vi "stop.vi"(8 "error in (no error)":errorcluster, 11 "references":T1) -> (0 "error out":errorcluster)   [LabVIEW 2015, in "lv-recipe-machine.lvlib"]
doc: "stop.vi will stop the asynchronously running main and de-allocate any internal resources."
uses:
  lv-recipe-machine.lvlib
  _controls/references.ctl
  _controls/change.ctl
  _controls/automatic_state.ctl
  _controls/manual_state.ctl
  _controls/mode.ctl
  _controls/status.ctl
  _controls/configuration.ctl
  _controls/recipe_step.ctl
  _controls/recipe_data.ctl
  _controls/data.ctl
  _controls/output.ctl
  _controls/input_command.ctl
  _controls/input.ctl
  _controls/transition.ctl
  _controls/timer.ctl
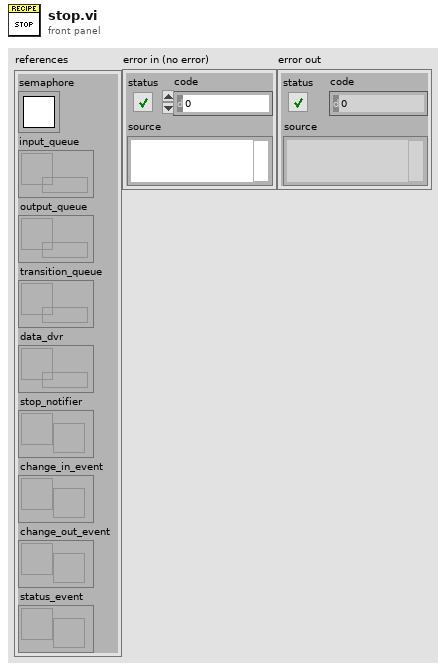
[diagram p1: front panel]
types:
  T1 = typedef "lv-recipe-machine.lvlib/references.ctl" = cluster{"semaphore":T2, "input_queue":refnum<queue>, "output_queue":refnum<queue>, "transition_queue":refnum<queue>, "data_dvr":refnum<data-value>, "stop_notifier":refnum<notifier>, "change_in_event":refnum<user-event>, "change_out_event":refnum<user-event>, "status_event":refnum<user-event>}
  T2 = typedef "Semaphore RefNum" = refnum<k1>
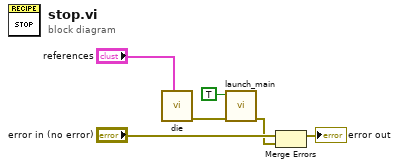
[diagram p0: block diagram]
diagram:
  n1 = call "die.vi"("references"="references") -> ("error out"=w3:errorcluster)  [unwired: 10 in]
  n2 = call "launch_main.vi"("error in (no error)"=w3, 11:TRUE ("Run(F)/Abort(T)")) -> ("error out"=w2:errorcluster)  [unwired: 8 in, 1 out]
  n3 = Merge Errors("error in (no error)", w2) -> (→"error out":errorcluster)
